vi "VG-verifyCalibrationPath.vi"(8 "error in (no error)":errorcluster, 11 "VG-VNA_GUI in":refnum<class "VG-VNA_GUI.lvclass">) -> (0 "error out":errorcluster, 2 "Valid?":bool, 3 "VG-VNA_GUI out":refnum<class "VG-VNA_GUI.lvclass">)   [LabVIEW 2020, in "VG-VNA_GUI.lvlib" / "VG-VNA_GUI.lvclass"]
uses:
  VG-VNA_GUI.lvclass
  VG-VNA_GUI.lvclass/VG-VNA_GUI.ctl
  <userlib>/_OpenG.lib/file/file.llb/Valid Path - Traditional__ogtk.vi
  <userlib>/_OpenG.lib/file/file.llb/openg_file.lvlib
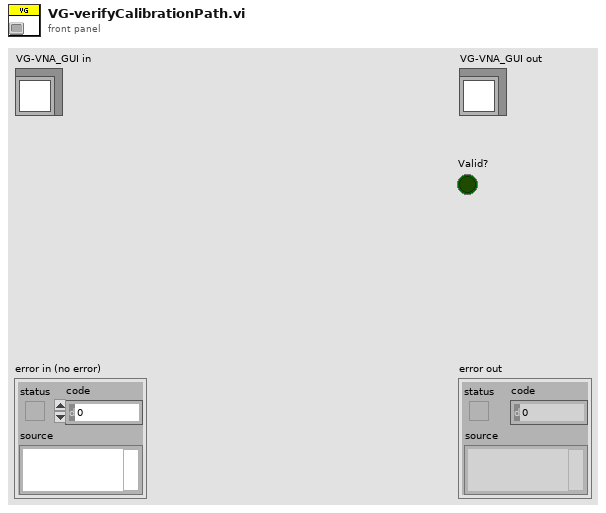
[diagram p1: front panel]
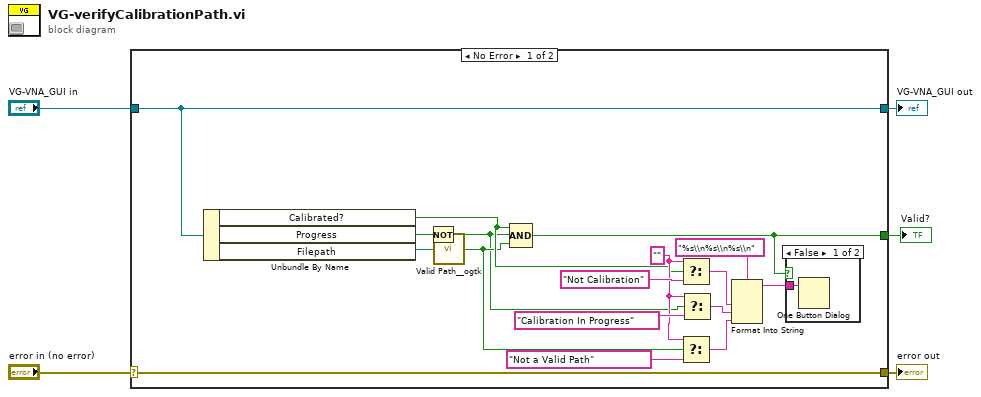
[diagram p0: block diagram]
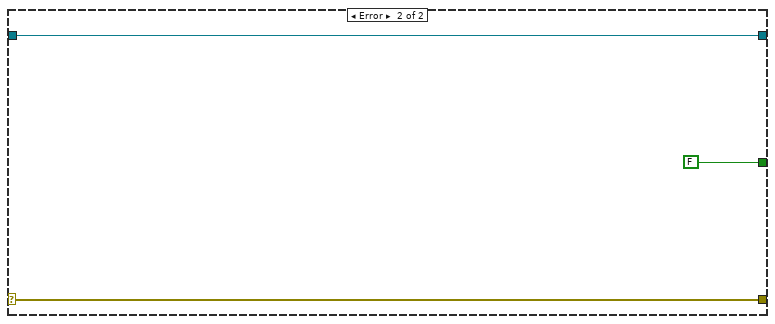
[diagram p3: hidden frame]
diagram:
  n1 = case shown="No Error" "error in (no error)" {
    selector: "error in (no error)" -> [w22 w26]
    tunnel: [w22 w26] -> w4
    tunnel: [w21 w25] -> w2
    tunnel: "VG-VNA_GUI in" -> [w21 w25]
    tunnel: [w11 FALSE] -> w1
    frame No Error {
      w17 = "" ("f")
      n2 = Unbundle By Name(w21) -> ("Calibrated?"=w15:bool, "Progress"=w14:bool, "Filepath"=w20:path)
      n3 = Not(x=w14) -> (.not. x?=w12:bool)
      n4 = call-poly <userlib>:"Valid Path__ogtk.vi"("path"=w20) -> ("valid"=w13:bool)
      n5 = Compound Arithmetic op=AND(w15, w12, w13) -> (w11:bool)
      n6 = Select(t=w17, s=w15, f="Not Calibration" ("input 1")) -> (s? t:f=w9:string)
      n7 = Select(t=w17, s=w13, f="Not a Valid Path" ("input 1")) -> (s? t:f=w7:string)
      n8 = Select(t=w17, s=w12, f="Calibration In Progress" ("input 1")) -> (s? t:f=w8:string)
      n9 = Format Into String(format string="%s\\n%s\\n%s\\n", w9, w8, w7) -> (resulting string=w6:string)  [unwired: 2 in, 1 out]
      n10 = case shown="False" w11 {
        tunnel: w6 -> [w23 _]
        frame False {
          n11 = One Button Dialog(message=w23) -> ()  [unwired: 1 in, 1 out]
        }
        frame True {
        }
      }
    }
    frame Error {
    }
  }
  "error out" <- w4
  "VG-VNA_GUI out" <- w2
  "Valid?" <- w1
